vi "degree_to_radian.vi"(1 "angle in":dbl[unit]) -> (0 "angle out":dbl[unit])   [LabVIEW 2010]
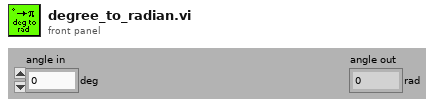
[diagram p1: front panel]
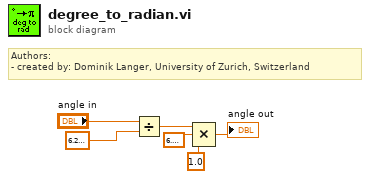
[diagram p0: block diagram]
diagram:
  # "Authors: \n- created by: Dominik Langer, University of Zurich, Switzerland"
  n1 = Divide(x="angle in", y=dbl[unit] 6.283185307179586) -> (x/y=w4:dbl)
  n2 = Compound Arithmetic op=MULTIPLY(w4, 6.283185307179586, dbl[unit] 1.0 ("value")) -> (→"angle out":dbl[unit])
